vi "Replace Diagram Contents.vi"(8 "error in (no error)":errorcluster, 10 "Template VI":path, 11 "Target VI":refnum<vi>) -> (0 "error out":errorcluster, 3 "dup Target VI":refnum<vi>)   [LabVIEW 2020, in "Message Rescripter.lvlib"]
uses:
  Message Rescripter.lvlib
  <vilib>/Utility/traverseref.llb/TRef TravTarget.ctl
  <vilib>/Utility/miscctls.llb/LVPointTypeDef.ctl
  <vilib>/Utility/traverseref.llb/VI Scripting - Traverse.lvlib
  MessageMakerProvider/AFPP Shared/AFPP Shared.lvlib
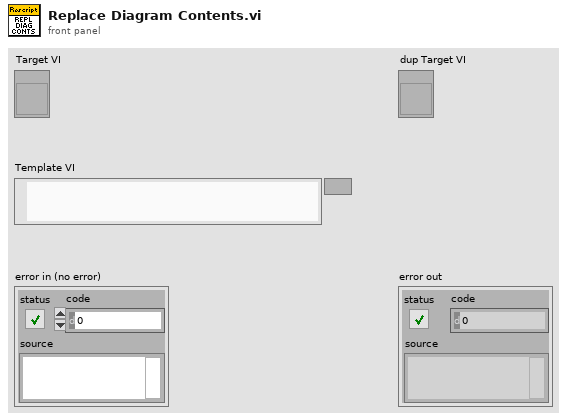
[diagram p1: front panel]
types:
  T1 = typedef "LVPointTypeDef.ctl" = cluster{"Horizontal":i16, "Vertical":i16}
  T2 = typedef "TRef TravTarget.ctl" = enum16{"FP", "BD", "Other"}
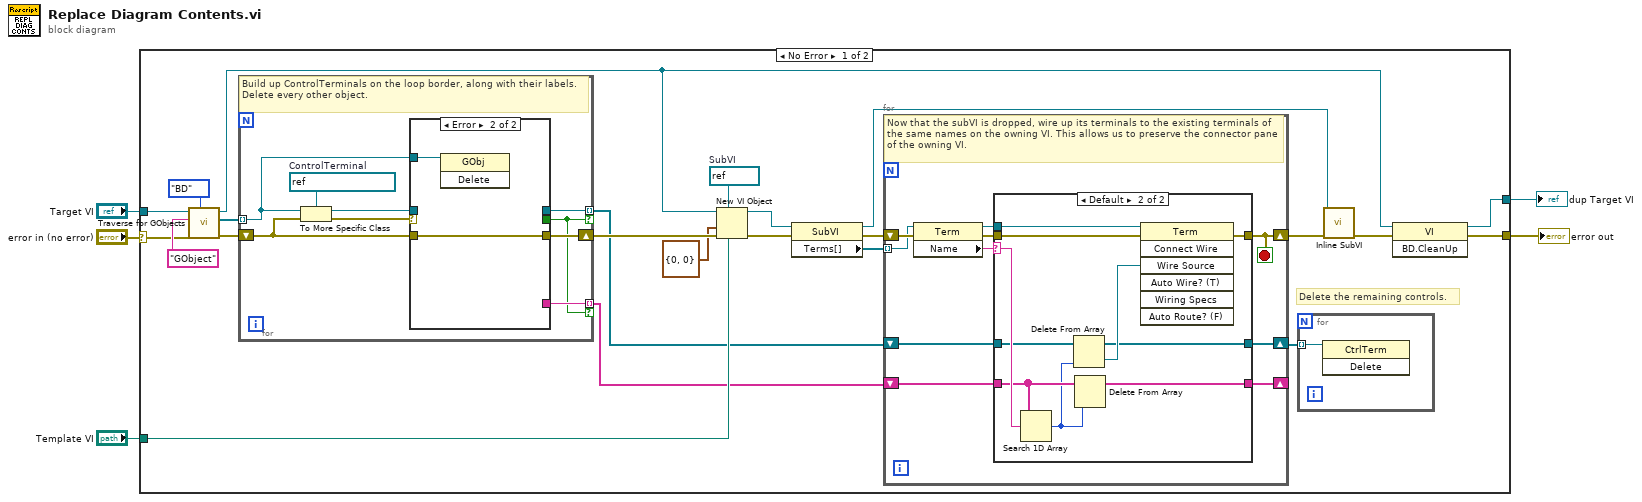
[diagram p0: block diagram]
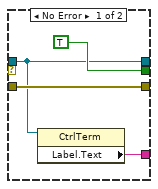
[diagram p3: hidden frame]
diagram:
  n1 = case shown="No Error" "error in (no error)" {
    selector: "error in (no error)" -> [w6 w69]
    tunnel: "Template VI" -> [w24 _]
    tunnel: [w23 w69] -> w4
    tunnel: "Target VI" -> [w22 w68]
    tunnel: [w9 w68] -> w2
    frame No Error {
      w18 = refnum<vi> refnum  # SubVI
      # "Delete the remaining controls."
      n2 = call <vilib>:"Traverse for GObjects.vi"("Traverse Target"=TRef_TravTarget."BD", "error in (no error)"=w6, "Class Name"="GObject", "VI Refnum"=w22) -> ("error out"=w26:errorcluster, "References"=w25:refnum<vi>[], "dup VI Refnum"=w8:refnum<vi>)  [unwired: 4 in, 1 out]
      n3 = for {
        tunnel: w25 -> [w57] mode=indexing
        tunnel: [w58] -> w20 mode=indexing if=w53
        shift-right: [w55] -> w21
        shift-left: w26 -> [w56]
        tunnel: [w54] -> w19 mode=indexing if=w53
        w61 = refnum<vi> refnum  # ControlTerminal
        # "Build up ControlTerminals on the loop border, along with their labels. Delete every other object."
        n4 = To More Specific Class(target class=w61, reference=w57, error in=w56) -> (specific class reference=w59:refnum<vi>, error out=w60:errorcluster)
        n5 = case shown="Error" w60 {
          tunnel: w59 -> [w63 _]
          tunnel: [w63 _] -> w58
          tunnel: [TRUE _] -> w53
          tunnel: w57 -> [_ w67]
          tunnel: w56 -> [w64 w66]
          tunnel: [w64 w66] -> w55
          tunnel: [w62 _] -> w54
          frame No Error {
            n6 = property class="CtrlTerm"(reference=w63) -> ("Label.Text"=w62:string)  [unwired: 1 in, 2 out]
          }
          frame Error {
            n7 = invoke class="GObj" method="Delete"(reference=w67) -> ()  [unwired: 2 in, 3 out]
          }
        }
      }
      n8 = New VI Object(vi object class=w18, owner refnum=w8, position/next to=T1 {"Horizontal"=0, "Vertical"=0} ("location"), 6:w24, 8:w21) -> (object refnum=w15:refnum<vi>, 0:w16:errorcluster)  [unwired: 3 in]
      n9 = property class="SubVI"(reference=w15, error in=w16) -> (reference out=w12:refnum<vi>, error out=w14:errorcluster, "Terms[]"=w13:refnum<vi>[])
      n10 = for {
        shift-right: [w32] -> w7
        shift-left: w14 -> [w39]
        tunnel: w13 -> [w38] mode=indexing
        shift-right: [w31] -> w11
        shift-left: w20 -> [w35]
        shift-right: [w30] -> _
        shift-left: w19 -> [w37]
        stop <- w32 stop-if-true
        # "Now that the subVI is dropped, wire up its terminals to the existing terminals of the same names on the owning VI. This allows us to preserve the connector pane of the owning VI."
        n11 = property class="Term"(reference=w38, error in=w39) -> (reference out=w33:refnum<vi>, error out=w34:errorcluster, "Name"=w36:string)
        n12 = case shown="Default" w36 {
          selector: w36 -> [_ w52]
          tunnel: w37 -> [w40 w45]
          tunnel: w35 -> [w41 w51]
          tunnel: w34 -> [w42 w50]
          tunnel: w33 -> [_ w49]
          tunnel: [w42 w48] -> w32
          tunnel: [w41 w46] -> w31
          tunnel: [w40 w43] -> w30
          frame "" {
          }
          frame Default {
            n13 = Search 1D Array(1D array=w45, element=w52) -> (index of element=w44:i32)  [unwired: 1 in]
            n14 = Delete From Array(array=w51, index=w44) -> (deleted portion=w47:refnum<vi>, array with subset deleted=w46:refnum<vi>[])  [unwired: 1 in]
            n15 = Delete From Array(array=w45, index=w44) -> (array with subset deleted=w43:string[])  [unwired: 1 in, 1 out]
            n16 = invoke class="Term" method="Connect Wire"(reference=w49, error in=w50, "Wire Source"=w47) -> (error out=w48:errorcluster)  [unwired: 4 in, 6 out]
          }
        }
      }
      n17 = for {
        tunnel: w11 -> [w29] mode=indexing
        n18 = invoke class="CtrlTerm" method="Delete"(reference=w29) -> ()  [unwired: 2 in, 3 out]
      }
      n19 = call "Inline SubVI.vi"("error in (no error)"=w7, "SubVI in"=w12) -> ("error out"=w10:errorcluster)  [unwired: 8 in, 1 out]
      n20 = invoke class="VI" method="BD.CleanUp"(reference=w8, error in=w10) -> (reference out=w9:refnum<vi>, error out=w23:errorcluster)  [unwired: 1 in, 1 out]
    }
    frame Error {
    }
  }
  "error out" <- w4
  "dup Target VI" <- w2
